vi "Error SenderSam.vi"(11 "queue in":refnum<queue>) -> ()   [LabVIEW 2014]
uses:
  controls/UI Data.ctl
  controls/Error Sender EnumSam.ctl
  controls/UI DataSam.ctl
  globals/RT Network Stream Endpoints.vi
  <resource>/objmgr/ni.dex.rc
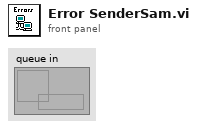
[diagram p1: front panel]
types:
  T1 = typedef "Error Sender EnumSam.ctl" = enum16{"Initialize", "Listen for Reader", "Send Error Messages"}
  T2 = typedef "UI DataSam.ctl" = cluster{"Message":string, "Data":variant}
  T3 = typedef "UI Data.ctl" = cluster{"Message":string, "Data":variant}
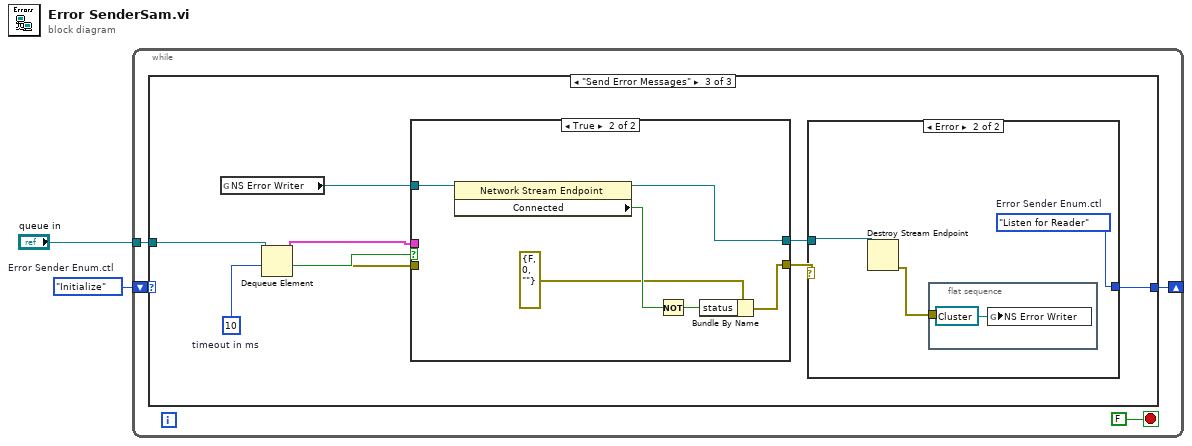
[diagram p0: block diagram]
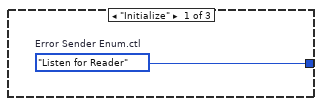
[diagram p2: hidden frame]
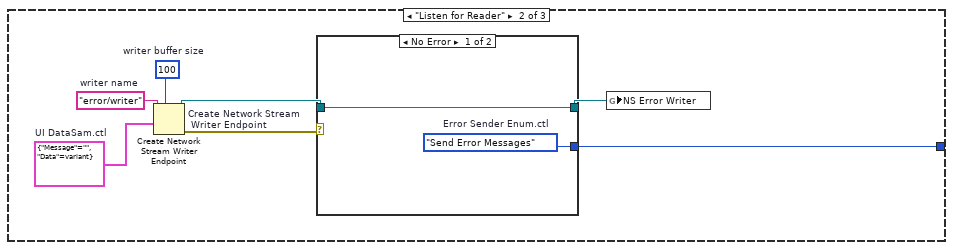
[diagram p3: hidden frame]
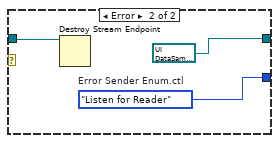
[diagram p4: hidden frame]
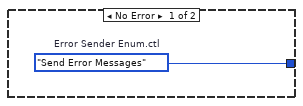
[diagram p5: hidden frame]
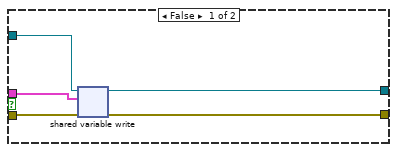
[diagram p6: hidden frame]
diagram:
  w2 = Error_Sender_EnumSam."Initialize"  # Error Sender Enum.ctl
  n1 = while {
    shift-right: [w6] -> _
    shift-left: w2 -> [w5]
    tunnel: "queue in" -> [w3]
    stop <- FALSE stop-if-true
    n2 = case shown="\"Send Error Messages\"" w5 {
      tunnel: [w7 w9 w21] -> w6
      tunnel: w3 -> [_ _ w28]
      frame "Initialize" {
        w7 = Error_Sender_EnumSam."Listen for Reader"  # Error Sender Enum.ctl
      }
      frame "Listen for Reader" {
        w12 = T2 {"Message"="", "Data"=variant}  # UI DataSam.ctl
        w13 = "error/writer"  # writer name
        w14 = 100  # writer buffer size
        n3 = Create Network Stream Writer Endpoint "Create Network Stream\n Writer Endpoint"(7:w14, 9:w12, 11:w13) -> (0:w10:errorcluster, 3:w11:refnum<k21>)  [unwired: 4 in]
        n4 = case shown="No Error" w10 {
          tunnel: w11 -> [w15 w19]
          tunnel: [w16 w18] -> w9
          tunnel: [w15 refnum<k21> refnum ("writer name")] -> w8
          frame No Error {
            w16 = Error_Sender_EnumSam."Send Error Messages"  # Error Sender Enum.ctl
          }
          frame Error {
            w18 = Error_Sender_EnumSam."Listen for Reader"  # Error Sender Enum.ctl
            n5 = Destroy Stream Endpoint(11:w19) -> ()  [unwired: 1 in, 1 out]
          }
        }
        n6 = global write "RT Network Stream Endpoints.vi" "NS Error Writer"(w8) -> ()
      }
      frame "Send Error Messages" {
        w27 = 10  # timeout in ms
        n7 = global read "RT Network Stream Endpoints.vi" "NS Error Writer"() -> (w25:refnum<k21>)
        n8 = Dequeue Element(queue=w28, timeout in ms (-1)=w27) -> (element=w23:T3, timed out?=w26:bool, error out=w24:errorcluster)  [unwired: 1 in, 1 out]
        n9 = case shown="True" w26 {
          tunnel: w25 -> [w38 w44]
          tunnel: w24 -> [w37 _]
          tunnel: w23 -> [w34 _]
          tunnel: [w36 w43] -> w20
          tunnel: [w35 w39] -> w22
          frame False {
            n10 = shared-variable-write(w38, w37, w34) -> (w36:refnum<k21>, w35:errorcluster)  [unwired: 1 in, 1 out]
          }
          frame True {
            n11 = property class="Network Stream Endpoint"(reference=w44) -> (reference out=w43:refnum<k21>, "Connected"=w42:bool)  [unwired: 1 in, 1 out]
            n12 = Not(x=w42) -> (.not. x?=w40:bool)
            n13 = Bundle By Name(cluster=errorcluster {"status"=FALSE, "code"=0, "source"=""} ("error IO"), "status"=w40) -> (w39:errorcluster)
          }
        }
        n14 = case shown="Error" w22 {
          tunnel: [w29 w30] -> w21
          tunnel: w20 -> [_ w32]
          frame No Error {
            w29 = Error_Sender_EnumSam."Send Error Messages"  # Error Sender Enum.ctl
          }
          frame Error {
            w30 = Error_Sender_EnumSam."Listen for Reader"  # Error Sender Enum.ctl
            n15 = Destroy Stream Endpoint(11:w32) -> (0:w31:errorcluster)  [unwired: 1 in]
            n16 = flat-sequence {
              tunnel: w31 -> [_]
              frame #0 {
                n17 = global write "RT Network Stream Endpoints.vi" "NS Error Writer"(refnum<k21> refnum ("NS Error Writer")) -> ()
              }
            }
          }
        }
      }
    }
  }
